vi "Main.vi"(11 "Module Admin":refnum<class "Delacor_lib_QMH_Module Admin.lvclass">) -> ()   [LabVIEW 2020, in "Rename as Top-Level Library.lvlib"]
doc: "This template is based off of the Queued Message Handler design pattern and the Queued Message Handler project template that ships with LabVIEW.\n\nThe main difference is that the queue is private to this module and communication between modules is performed via Broadcast and Request events.\n\nRequest events are wrapped in public API methods and are handled in the Event Handling Loop (EHL) of this VI. Any module can register for Broadcast events sent by this module. The EHL generates messages based on user interface actions.\n\nThe Message Handling Loop (MHL) processes messages generated by the EHL, or by other messages. The messages are string values, so new messages can be added easily to the Message Cases case structure in the MHL. Each message cluster can also provide an optional value for Message Data, which is a variant that can be converted to whatever message-specific data is required.\n_____\nBased on DQMH Project Template 6.1.0.94."
uses:
  Rename as Top-Level Library.lvlib
  <vilib>/Delacor/Delacor QMH/Libraries/Module Admin_class/Delacor_lib_QMH_Module Admin.lvclass
  Module Data--cluster.ctl
  <vilib>/Delacor/Delacor QMH/Libraries/Message Queue_class/Delacor_lib_QMH_Message Queue.lvclass/Delacor_lib_QMH_Message Queue.ctl
  Stop Argument--cluster.ctl
  <vilib>/Utility/miscctls.llb/LVPointTypeDef.ctl
  <vilib>/Delacor/Delacor QMH/Libraries/Module Admin_class/Delacor_lib_QMH_Module Admin.lvclass/Delacor_lib_QMH_Module Admin.ctl
  <vilib>/Delacor/Delacor QMH/Libraries/Message Queue_class/Delacor_lib_QMH_Enqueue Message (Single).vi
  <vilib>/Delacor/Delacor QMH/Libraries/Module Admin_class/Delacor_lib_QMH_Get External Launch.vi
  <vilib>/Utility/error.llb/Error Cluster From Error Code.vi
  <vilib>/ErrorRing/Error Ring.xnode
  <vilib>/Delacor/Delacor QMH/Libraries/Message Queue_class/Delacor_lib_QMH_Message Queue.lvclass
  <vilib>/Peloton/Pelobuttons/Pelobuttons_lib_Pelobuttons.lvlib
panel:
  out "error out":errorcluster
  out "Status":string
  in  "Simulate MHL Error":bool
  in  "Simulate EHL Error":bool
  # "Make sure you use Pelobuttons to edit your Main UI"
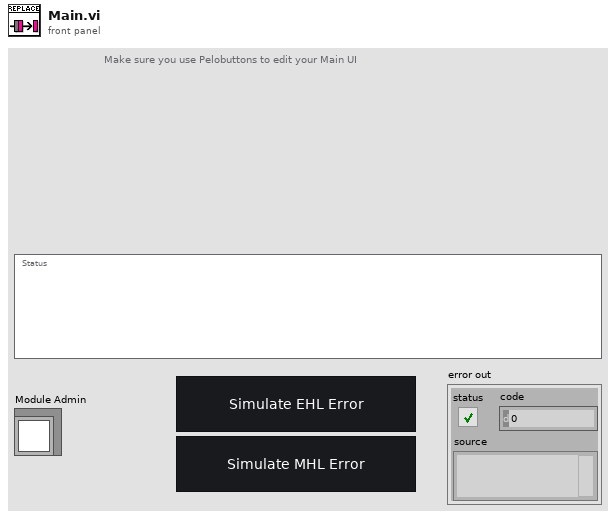
[diagram p1: front panel]
types:
  T1 = typedef "Rename as Top-Level Library.lvlib/Request Events--cluster.ctl" = cluster{"Stop Module":refnum<user-event>, "Show Panel":refnum<user-event>, "Hide Panel":refnum<user-event>, "Get Module Execution Status":refnum<user-event>, "Show Diagram":refnum<user-event>}
  T2 = typedef "Rename as Top-Level Library.lvlib/Module Data--cluster.ctl" = cluster{"Status":string}
  T3 = enum32{"invalid lock state", "Not Locked", "Locked (No Password)", "Password-protected"}
  T4 = typedef "Rename as Top-Level Library.lvlib/Stop Argument--cluster.ctl" = cluster{"Origin":string, "Exit via Stop Module Req?":bool, "Wait for Module to stop?":bool}
  T5 = typedef "LVPointTypeDef.ctl" = cluster{"Horizontal":i16, "Vertical":i16}
  T6 = enum32{"Invalid", "Standard", "Closed", "Hidden", "Minimized", "Maximized"}
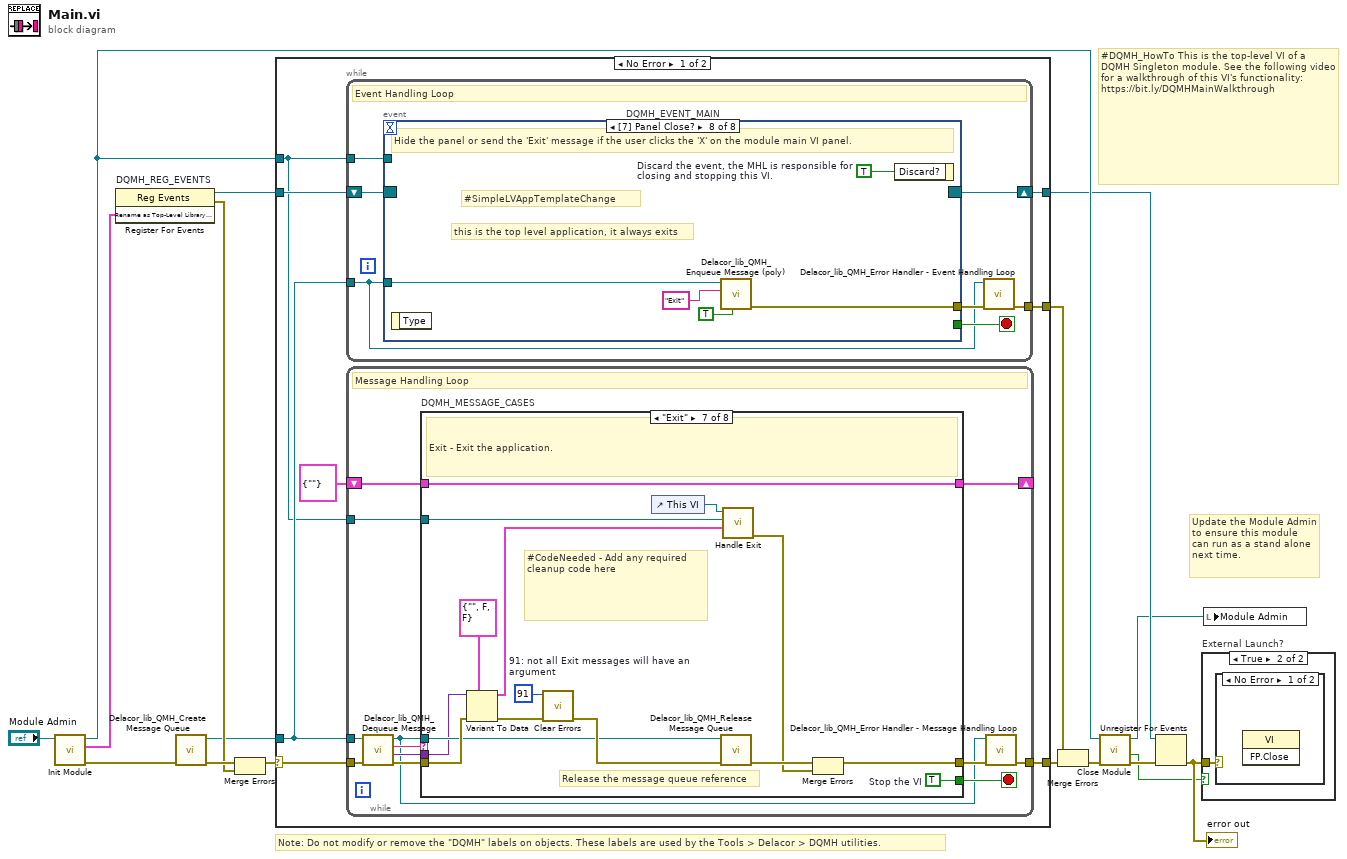
[diagram p0: block diagram]
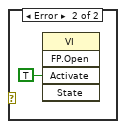
[diagram p3: hidden frame]
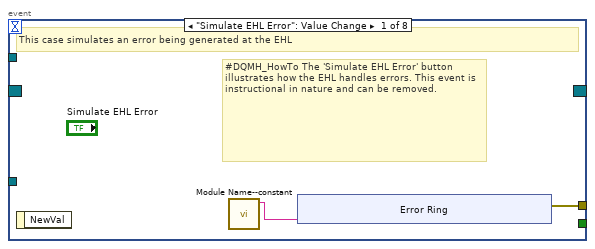
[diagram p4: hidden frame]
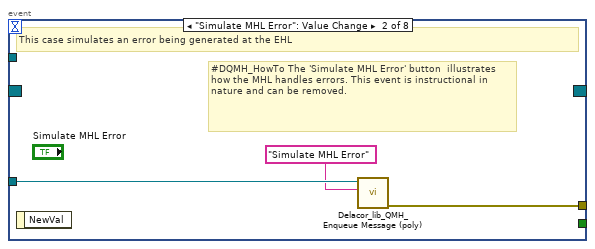
[diagram p5: hidden frame]
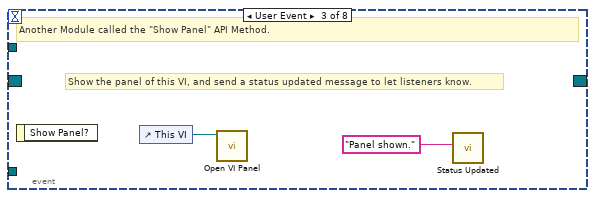
[diagram p6: hidden frame]
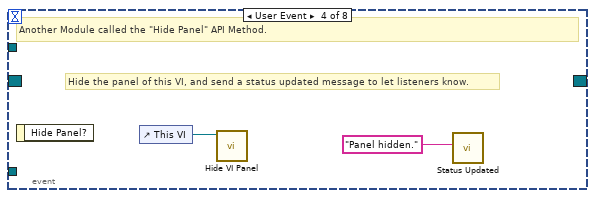
[diagram p7: hidden frame]
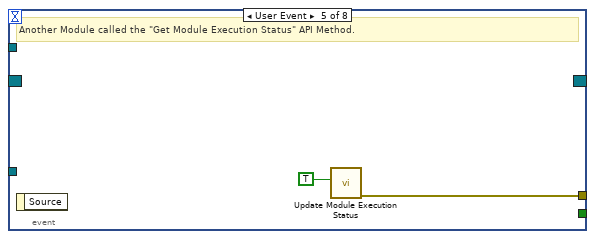
[diagram p8: hidden frame]
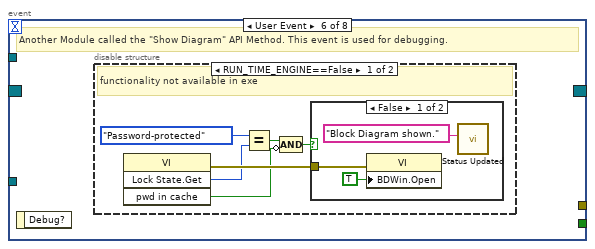
[diagram p9: hidden frame]
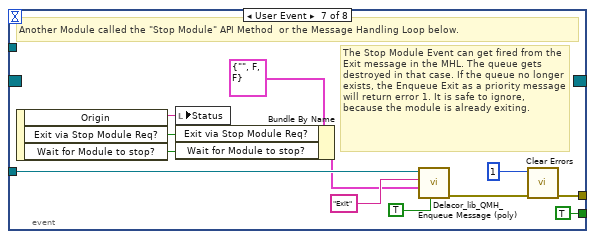
[diagram p12: hidden frame]
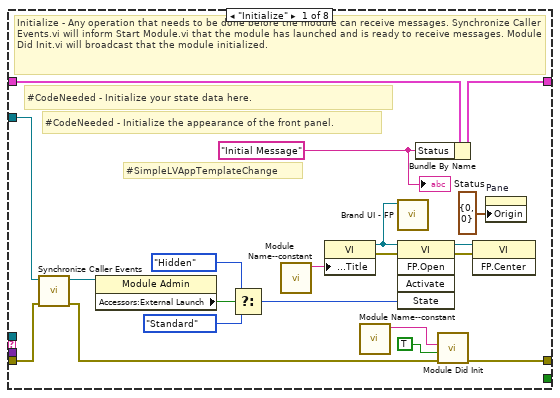
[diagram p13: hidden frame]
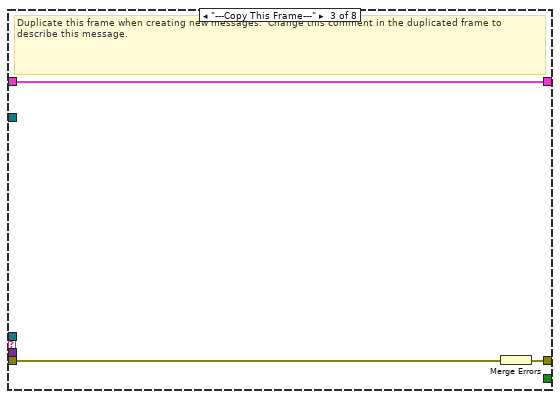
[diagram p15: hidden frame]
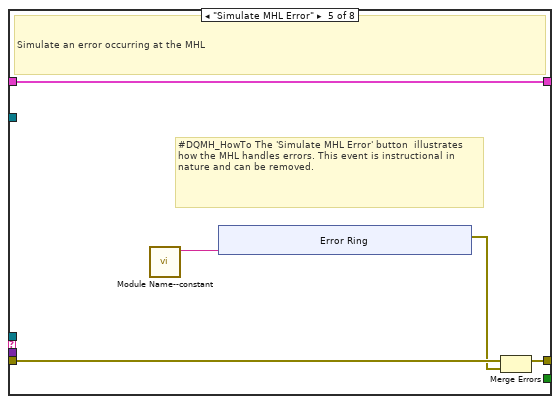
[diagram p17: hidden frame]
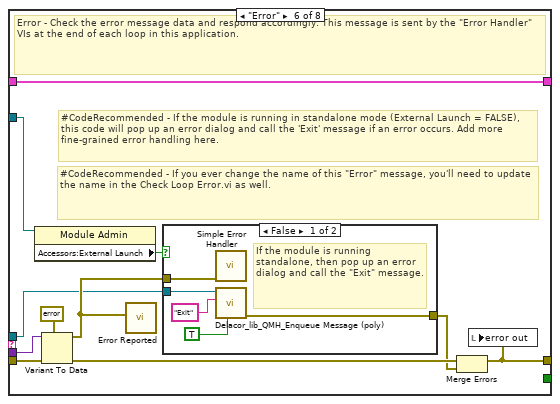
[diagram p18: hidden frame]
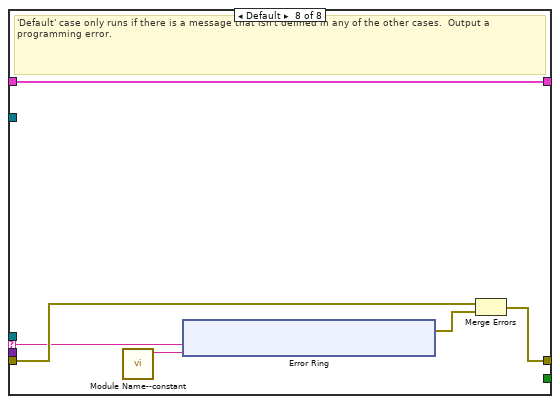
[diagram p20: hidden frame]
diagram:
  # "#DQMH_HowTo This is the top-level VI of a DQMH Singleton module. See the following video for a walkthrough of this VI's functionality: https://bit.ly/DQMHMainWalkthrough"
  # "Note: Do not modify or remove the \"DQMH\" labels on objects. These labels are used by the Tools > Delacor > DQMH utilities."
  # "Update the Module Admin to ensure this module can run as a stand alone next time."
  n1 = call "Init Module.vi"("Singleton Module Admin in"="Module Admin") -> ("error out"=w16:errorcluster, "Rename as Top-Level Library Request Events"=w5:T1, "Singleton Module Admin out"=w8:refnum<class "Delacor_lib_QMH_Module Admin.lvclass">)  [unwired: 8 in]
  n2 = register-events "DQMH_REG_EVENTS"(w5) -> (reference out=w6:refnum<event-registration>, error out=w9:errorcluster)  [unwired: 2 in]
  n3 = call <vilib>:"Delacor_lib_QMH_Create Message Queue.vi"("error in"=w16) -> ("error out"=w11:errorcluster, "Message Queue"=w4:refnum<class "Delacor_lib_QMH_Message Queue.lvclass">)  [unwired: 9 in]
  n4 = Merge Errors(w11, w9) -> (w10:errorcluster)
  n5 = case shown="No Error" w10 {
    selector: w10 -> [w23 w175]
    tunnel: [w25 w174] -> w17
    tunnel: [w22 w180] -> w7
    tunnel: w6 -> [w20 w180]
    tunnel: w4 -> [w19 w173]
    tunnel: [w24 _] -> w14
    tunnel: w8 -> [w18 w176]
    frame No Error {
      n6 = while {
        tunnel: w19 -> [w26]
        shift-right: [w29] -> w22
        shift-left: w20 -> [w30]
        tunnel: [w31] -> w24
        tunnel: w18 -> [w27]
        stop <- w28 stop-if-true
        # "Event Handling Loop"
        n7 = event "DQMH_EVENT_MAIN" shown="[7] Panel Close?" {
          selector: w30 -> [_ _ _ _ _ _ _ _]
          dyn-events: [_ _ _ _ _ _ _ _] -> w29
          timeout: _ -> [_ _ _ _ _ _ _ _]
          tunnel: [_ _ _ _ _ _ TRUE ("Discard?") _] -> w28
          tunnel: w26 -> [_ w43 _ _ _ _ w67 w74]
          tunnel: [w34 w44 _ _ w50 _ w70 w76] -> w32
          tunnel: w27 -> [_ _ _ _ _ _ _ _]
          event "Simulate EHL Error": Value Change {
            # "#DQMH_HowTo The 'Simulate EHL Error' button  illustrates how the EHL handles errors. This event is instructional in nature and can be removed."
            # "This case simulates an error being generated at the EHL"
            n8 = event-data() -> ()  [unwired: 1 in, 1 out]
            n9 = call "Module Name--constant.vi"() -> ("Module Name"=w33:string)  [unwired: 11 in]
            n10 = xnode "Error Ring"("parameter 0"=w33) -> ("error out"=w34:errorcluster)
          }
          event "Simulate MHL Error": Value Change {
            # "#DQMH_HowTo The 'Simulate MHL Error' button  illustrates how the MHL handles errors. This event is instructional in nature and can be removed."
            # "This case simulates an error being generated at the EHL"
            n11 = event-data() -> ()  [unwired: 1 in, 1 out]
            n12 = call-poly <vilib>:"Delacor_lib_QMH_Enqueue Message (poly).vi"("Message"="Simulate MHL Error", "Message Queue in"=w43) -> ("error out"=w44:errorcluster)  [unwired: 8 in, 1 out]
          }
          event User Event {
            # "Show the panel of this VI, and send a status updated message to let listeners know."
            # "Another Module called the \"Show Panel\" API Method."
            n13 = event-data() -> ()  [unwired: 1 in, 1 out]
            n14 = control-ref of="This VI"() -> (w46:refnum<vi>)
            n15 = call "Open VI Panel.vi"("VI"=w46) -> ()  [unwired: 10 in, 1 out]
            n16 = call "Status Updated.vi"("Status"="Panel shown." ("format string")) -> ()  [unwired: 10 in, 1 out]
          }
          event User Event {
            # "Hide the panel of this VI, and send a status updated message to let listeners know."
            # "Another Module called the \"Hide Panel\" API Method."
            n17 = event-data() -> ()  [unwired: 1 in, 1 out]
            n18 = control-ref of="This VI"() -> (w48:refnum<vi>)
            n19 = call "Hide VI Panel.vi"("VI"=w48) -> ()  [unwired: 10 in, 1 out]
            n20 = call "Status Updated.vi"("Status"="Panel hidden." ("format string")) -> ()  [unwired: 10 in, 1 out]
          }
          event User Event {
            # "Another Module called the \"Get Module Execution Status\" API Method."
            n21 = event-data() -> ()  [unwired: 1 in, 1 out]
            n22 = call "Update Module Execution Status.vi"("Running?"=TRUE) -> ("error out"=w50:errorcluster)  [unwired: 10 in]
          }
          event User Event {
            # "Another Module called the \"Show Diagram\" API Method. This event is used for debugging."
            n23 = event-data() -> ()  [unwired: 1 in, 1 out]
            n24 = disable-structure shown="RUN_TIME_ENGINE==False" {
              frame condition #0 (active) {
                # "functionality not available in exe"
                n25 = invoke class="VI" method="Lock State.Get"() -> (error out=w56:errorcluster, "Get Lock State"=w55:T3, "pwd in cache"=w52:bool)  [unwired: 4 in, 1 out]
                n26 = Equal?(x=T3."Password-protected", y=w55) -> (x = y?=w53:bool)
                n27 = Compound Arithmetic op=AND(w53, invert w52) -> (w51:bool)
                n28 = case shown="False" w51 {
                  tunnel: w56 -> [w59 _]
                  frame False {
                    n29 = property class="VI"(error in=w59, "BDWin.Open"=TRUE ("Block Diagram Window:Open")) -> ()  [unwired: 1 in, 2 out]
                    n30 = call "Status Updated.vi"("Status"="Block Diagram shown." ("format string")) -> ()  [unwired: 10 in, 1 out]
                  }
                  frame True {
                    # "Password-protected VI, and the password is not in the cache. Do not show the diagram."
                  }
                }
              }
              frame condition #1 {
              }
            }
          }
          event User Event {
            # "The Stop Module Event can get fired from the Exit message in the MHL. The queue gets destroyed in that case. If the queue no longer exists, the Enqueue Exit as a priority message will return error 1. It is safe to ignore, because the module is already exiting."
            # "Another Module called the \"Stop Module\" API Method  or the Message Handling Loop below."
            n31 = event-data() -> ("Origin"=w66:string, "Exit via Stop Module Req?"=w62:bool, "Wait for Module to stop?"=w61:bool)  [unwired: 1 in]
            n32 = local write "Status"(w66) -> ()
            n33 = Bundle By Name(cluster=T4 {"Origin"="", "Exit via Stop Module Req?"=FALSE, "Wait for Module to stop?"=FALSE} ("Stop Argument"), "Exit via Stop Module Req?"=w62, "Wait for Module to stop?"=w61) -> (w60:T4)
            n34 = call-poly <vilib>:"Delacor_lib_QMH_Enqueue Message (poly).vi"("Priority Message? (F)"=TRUE, "Message Data"=w60, "Message"="Exit", "Message Queue in"=w67) -> ("error out"=w71:errorcluster)  [unwired: 6 in, 1 out]
            n35 = call <vilib>:"Clear Errors.vi"("error in (no error)"=w71, "specific error code to clear (0: all)"=1) -> ("error out"=w70:errorcluster)  [unwired: 4 in, 1 out]
          }
          event Panel Close? {
            w75 = TRUE  # Discard the event, the MHL is responsible for closing and stopping this VI.
            # "#SimpleLVAppTemplateChange"
            # "this is the top level application, it always exits"
            # "Hide the panel or send the 'Exit' message if the user clicks the 'X' on the module main VI panel."
            n36 = event-data() -> ()  [unwired: 1 in, 1 out]
            n37 = call-poly <vilib>:"Delacor_lib_QMH_Enqueue Message (poly).vi"("Priority Message? (F)"=TRUE, "Message"="Exit", "Message Queue in"=w74) -> ("error out"=w76:errorcluster)  [unwired: 7 in, 1 out]
            n38 = event-data("Discard?"=w75) -> ()  [unwired: 1 in, 1 out]
          }
        }
        n39 = call-dynamic "Delacor_lib_QMH_Error Handler - Event Handling Loop.vi"("error in"=w32, "Message Queue in"=w26) -> ("dup error in"=w31:errorcluster)  [unwired: 8 in, 1 out]
      }
      n40 = while {
        tunnel: w19 -> [w79]
        shift-right: [w83] -> _
        shift-left: T2 {"Status"=""} ("Data Cluster") -> [w84]
        tunnel: w23 -> [w87]
        tunnel: [w85] -> w25
        tunnel: w18 -> [w77]
        stop <- w82 stop-if-true
        # "Message Handling Loop"
        n41 = call-dynamic "Delacor_lib_QMH_Dequeue Message.vi"("error in"=w87, "Message Queue in"=w79) -> ("error out"=w86:errorcluster, "Message Data"=w80:variant, "Message"=w81:string, "Message Queue out"=w78:refnum<class "Delacor_lib_QMH_Message Queue.lvclass">)  [unwired: 6 in]
        n42 = case "DQMH_MESSAGE_CASES" shown="\"Exit\"" w81 {
          selector: w81 -> [_ _ _ _ _ _ _ w160]
          tunnel: w78 -> [_ _ _ _ _ w130 w152 _]
          tunnel: w86 -> [w106 w110 w113 w115 w120 w137 w158 w162]
          tunnel: [w104 w110 w112 w115 w119 w133 w155 w163] -> w88
          tunnel: w84 -> [w96 w109 w111 w114 w117 w132 w151 w161]
          tunnel: [w95 w109 w111 w114 w117 w132 w151 w161] -> w83
          tunnel: [_ _ _ _ _ _ w150 _] -> w82
          tunnel: w80 -> [_ _ _ _ _ w131 w149 _]
          tunnel: w77 -> [w97 _ _ _ _ w129 w144 _]
          frame "Initialize" {
            w91 = "Initial Message" ("Initial Message")
            # "#SimpleLVAppTemplateChange"
            # "#CodeNeeded - Initialize the appearance of the front panel."
            # "#CodeNeeded - Initialize your state data here."
            # "Initialize - Any operation that needs to be done before the module can receive messages. Synchronize Caller Events.vi will inform Start Module.vi that the module has launched and is ready to receive messages. Module Did Init.vi will broadcast that the module initialized."
            n43 = call "Synchronize Caller Events.vi"("error in (no error)"=w106, "Singleton Module Admin in"=w97) -> ("error out"=w105:errorcluster, "Singleton Module Admin out"=w92:refnum<class "Delacor_lib_QMH_Module Admin.lvclass">)  [unwired: 8 in]
            n44 = property class="Module Admin"(reference=w92) -> ("Accessors:External Launch"=w101:bool)  [unwired: 1 in, 2 out]
            n45 = Select(t=T6."Hidden" ("State"), s=w101, f=T6."Standard" ("State")) -> (s? t:f=w98:T6)
            n46 = call "Module Name--constant.vi"() -> ("Module Name"=w103:string)  [unwired: 11 in]
            n47 = property class="VI"("Front Panel.Title"=w103) -> (reference out=w89:refnum<vi>, error out=w108:errorcluster)  [unwired: 2 in]
            n48 = call "Module Name--constant.vi"() -> ("Module Name"=w93:string)  [unwired: 11 in]
            n49 = call <vilib>:"Brand UI - FP.vi"("VI Refnum (VI Caller If Empty)"=w89) -> ()  [unwired: 11 in]
            n50 = invoke class="VI" method="FP.Open"(reference=w89, error in=w108, "State"=w98) -> (reference out=w102:refnum<vi>, error out=w107:errorcluster)  [unwired: 2 in, 3 out]
            n51 = Bundle By Name(cluster=w96, "Status"=w91) -> (w95:T2)
            n52 = call "Module Did Init.vi"("error in (no error)"=w105, "Initialized?"=TRUE, "Origin"=w93) -> ("error out"=w104:errorcluster)  [unwired: 8 in]
            n53 = invoke class="VI" method="FP.Center"(reference=w102, error in=w107) -> ()  [unwired: 1 in, 3 out]
            n54 = property on="Pane" class="Pane"("Origin"=T5 {"Horizontal"=0, "Vertical"=0}) -> ()  [unwired: 2 in, 2 out]
            "Status" <- w91
          }
          frame "---Module Specific---" {
            # "Separator -- The following cases handle messages specific to this Module."
          }
          frame "---Copy This Frame---" {
            # "Duplicate this frame when creating new messages.  Change this comment in the duplicated frame to describe this message."
            n55 = Merge Errors(w113) -> (w112:errorcluster)
          }
          frame "---Exit and Error Handling---" {
            # "Separator - The following cases handle errors and exit messages."
          }
          frame "Simulate MHL Error" {
            # "#DQMH_HowTo The 'Simulate MHL Error' button  illustrates how the MHL handles errors. This event is instructional in nature and can be removed."
            # "Simulate an error occurring at the MHL"
            n56 = call "Module Name--constant.vi"() -> ("Module Name"=w116:string)  [unwired: 11 in]
            n57 = xnode "Error Ring"("parameter 0"=w116) -> ("error out"=w118:errorcluster)
            n58 = Merge Errors(w120, w118) -> (w119:errorcluster)
          }
          frame "Error" {
            # "#CodeRecommended - If you ever change the name of this \"Error\" message, you'll need to update the name in the Check Loop Error.vi as well."
            # "#CodeRecommended - If the module is running in standalone mode (External Launch = FALSE), this code will pop up an error dialog and call the 'Exit' message if an error occurs. Add more fine-grained error handling here."
            # "Error - Check the error message data and respond accordingly. This message is sent by the \"Error Handler\" VIs at the end of each loop in this application."
            n59 = property class="Module Admin"(reference=w129) -> ("Accessors:External Launch"=w128:bool)  [unwired: 1 in, 2 out]
            n60 = Variant To Data(error in=w137, type=errorcluster {"status"=FALSE, "code"=0, "source"=""} ("error constant"), Variant=w131) -> (data=w138:errorcluster, error out=w135:errorcluster)
            n61 = call "Error Reported.vi"("Error"=w138) -> ()  [unwired: 10 in, 1 out]
            n62 = case shown="False" w128 {
              tunnel: [w143 _] -> w134
              tunnel: w130 -> [w141 _]
              tunnel: w138 -> [w142 _]
              frame False {
                # "If the module is running standalone, then pop up an error dialog and call the \"Exit\" message."
                n63 = call <vilib>:"Simple Error Handler.vi"("error in (no error)"=w142) -> ()  [unwired: 4 in, 5 out]
                n64 = call-poly <vilib>:"Delacor_lib_QMH_Enqueue Message (poly).vi"("Priority Message? (F)"=TRUE, "Message"="Exit", "Message Queue in"=w141) -> ("error out"=w143:errorcluster)  [unwired: 7 in, 1 out]
              }
              frame True {
                # "If the module was launched externally, calling the Error Reported broadcast VI is the only action performed by the \"Error\" message. The module's caller can then process the error appropriately."
              }
            }
            n65 = Merge Errors(w135, w134) -> (w133:errorcluster)
            n66 = local write "error out"(w133) -> ()
          }
          frame "Exit" {
            w148 = 91  # 91: not all Exit messages will have an argument
            w150 = TRUE  # Stop the VI
            # "Release the message queue reference"
            # "#CodeNeeded - Add any required cleanup code here"
            # "Exit - Exit the application."
            n67 = Variant To Data(error in=w158, type=T4 {"Origin"="", "Exit via Stop Module Req?"=FALSE, "Wait for Module to stop?"=FALSE} ("Stop Argument"), Variant=w149) -> (data=w146:T4, error out=w154:errorcluster)
            n68 = call <vilib>:"Clear Errors.vi"("error in (no error)"=w154, "specific error code to clear (0: all)"=w148) -> ("error out"=w157:errorcluster)  [unwired: 4 in, 1 out]
            n69 = control-ref of="This VI"() -> (w145:refnum<vi>)
            n70 = call-dynamic "Delacor_lib_QMH_Release Message Queue.vi"("error in"=w157, "Message Queue"=w152) -> ("error out"=w156:errorcluster)  [unwired: 9 in]
            n71 = call "Handle Exit.vi"("Stop Argument"=w146, "Admin in"=w144, "VI reference"=w145) -> ("error out"=w153:errorcluster)  [unwired: 7 in, 1 out]
            n72 = Merge Errors(w156, w153) -> (w155:errorcluster)
          }
          frame Default {
            # "'Default' case only runs if there is a message that isn't defined in any of the other cases.  Output a programming error."
            n73 = call "Module Name--constant.vi"() -> ("Module Name"=w159:string)  [unwired: 11 in]
            n74 = xnode "Error Ring"("parameter 0"=w160, "parameter 1"=w159) -> ("error out"=w164:errorcluster)
            n75 = Merge Errors(w162, w164) -> (w163:errorcluster)
          }
        }
        n76 = call-dynamic "Delacor_lib_QMH_Error Handler - Message Handling Loop.vi"("error in"=w88, "Message Queue in"=w78) -> ("dup error in"=w85:errorcluster)  [unwired: 8 in, 1 out]
      }
    }
    frame Error {
      # "Synchronize Caller Events.vi will inform Start Module.vi that the module has launched and will let the code calling Start Module.vi register for broadcasts and would permit the caller receive the broadcast that an error occurred at launch time."
      n77 = call-dynamic "Delacor_lib_QMH_Release Message Queue.vi"("error in"=w175, "Message Queue"=w173) -> ("error out"=w174:errorcluster)  [unwired: 9 in]
      n78 = call "Synchronize Caller Events.vi"("Singleton Module Admin in"=w176) -> ("error out"=w181:errorcluster)  [unwired: 9 in, 1 out]
      n79 = call "Module Name--constant.vi"() -> ("Module Name"=w179:string)  [unwired: 11 in]
      n80 = Format Into String(format string="An error occurred during initialization. %s is no longer running.", w179) -> (resulting string=w177:string)  [unwired: 2 in, 1 out]
      n81 = Merge Errors(w174, w181) -> (w182:errorcluster)
      n82 = call "Error Reported.vi"("Additional Information"=w177, "Error"=w182) -> ()  [unwired: 9 in, 1 out]
    }
  }
  n83 = Merge Errors(w14, w17) -> (w13:errorcluster)
  n84 = call "Close Module.vi"("error in (no error)"=w13, "Module Admin in"=w8) -> ("error out"=w15:errorcluster, "External Launch"=w1:bool, "Module Admin out"=w2:refnum<class "Delacor_lib_QMH_Module Admin.lvclass">)  [unwired: 7 in]
  n85 = Unregister For Events(event registration refnum=w7, error in=w15) -> (error out=w12:errorcluster)
  "error out" <- w12
  n86 = case "External Launch?" shown="True" w1 {
    tunnel: w12 -> [_ w183]
    frame False {
    }
    frame True {
      n87 = case shown="No Error" w183 {
        frame No Error {
          n88 = invoke class="VI" method="FP.Close"() -> ()  [unwired: 3 in, 3 out]
        }
        frame Error {
          n89 = invoke class="VI" method="FP.Open"("Activate"=TRUE ("Activate?")) -> ()  [unwired: 4 in, 5 out]
        }
      }
    }
  }
  n90 = local write "Module Admin"(w2) -> ()
